vi "Read State.vi"(8 "error in (no error)":errorcluster, 11 "Expansion in":refnum<class "Expansion.lvclass">) -> (0 "error out":errorcluster, 2 "State":T1, 3 "Expansion out":refnum<class "Expansion.lvclass">)   [LabVIEW 2017, in "Expansion.lvclass"]
uses:
  Expansion.lvclass
  Type Defs/Expansion State.ctl
  Expansion.lvclass/Expansion.ctl
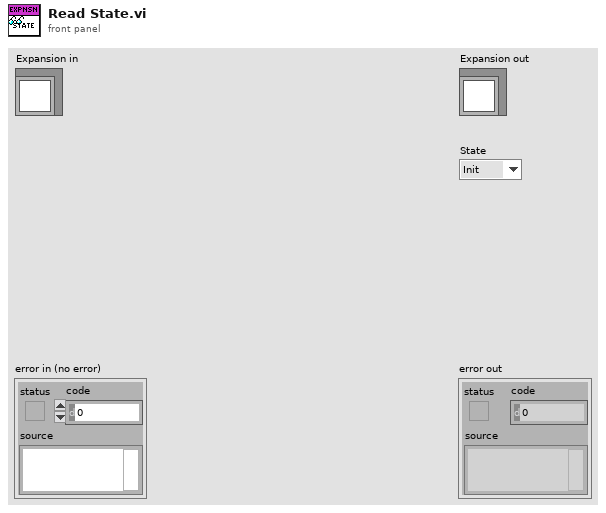
[diagram p1: front panel]
types:
  T1 = typedef "Expansion.lvclass/Expansion State.ctl" = enum16{"Init", "Update", "Go", "Move from Load to Heating", "Stop Motor", "Operate Cylinders", "Wait and Monitor", "Move from Heating to Unload", "Unload", "Move from Unload to Heating", "Move from Heating to Load", "Complete Process", "Stop", "Idle", "Error", "Shutdown"}
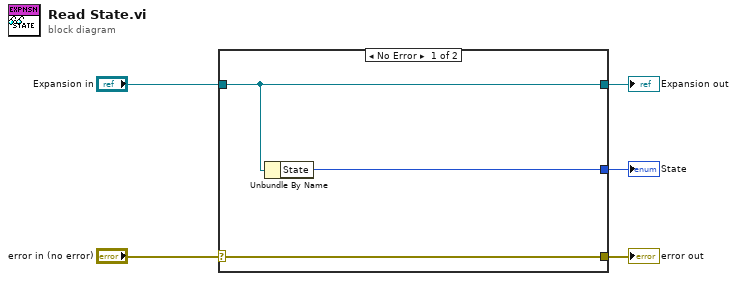
[diagram p0: block diagram]
diagram:
  n1 = case shown="No Error" "error in (no error)" {
    selector: "error in (no error)" -> [w8 w9]
    tunnel: [w8 w9] -> w4
    tunnel: [w7 w10] -> w2
    tunnel: "Expansion in" -> [w7 w10]
    tunnel: [w6 _] -> w1
    frame No Error {
      n2 = Unbundle By Name(w7) -> ("State"=w6:T1)
    }
    frame Error {
    }
  }
  "error out" <- w4
  "Expansion out" <- w2
  "State" <- w1
